vi "General Setting.vi"() -> ()   [LabVIEW 2020, in "Setting Lib.lvlib"]
uses:
  Setting Lib.lvlib
  Database Lib.lvlib
panel:
  in  "Frame Rate":u8=1 min=1 max=5 step=1
  in  "Threshold 5":dbl format="%#.1f"
  in  "Threshold 4":dbl format="%#.1f"
  in  "Threshold 3":dbl format="%#.1f"
  in  "Threshold 2":dbl format="%#.1f"
  in  "Threshold 1":dbl format="%#.1f"
  in  "Close":bool
  # "General Settings"
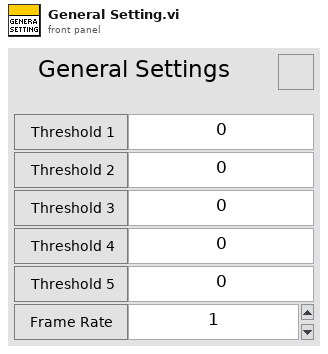
[diagram p1: front panel]
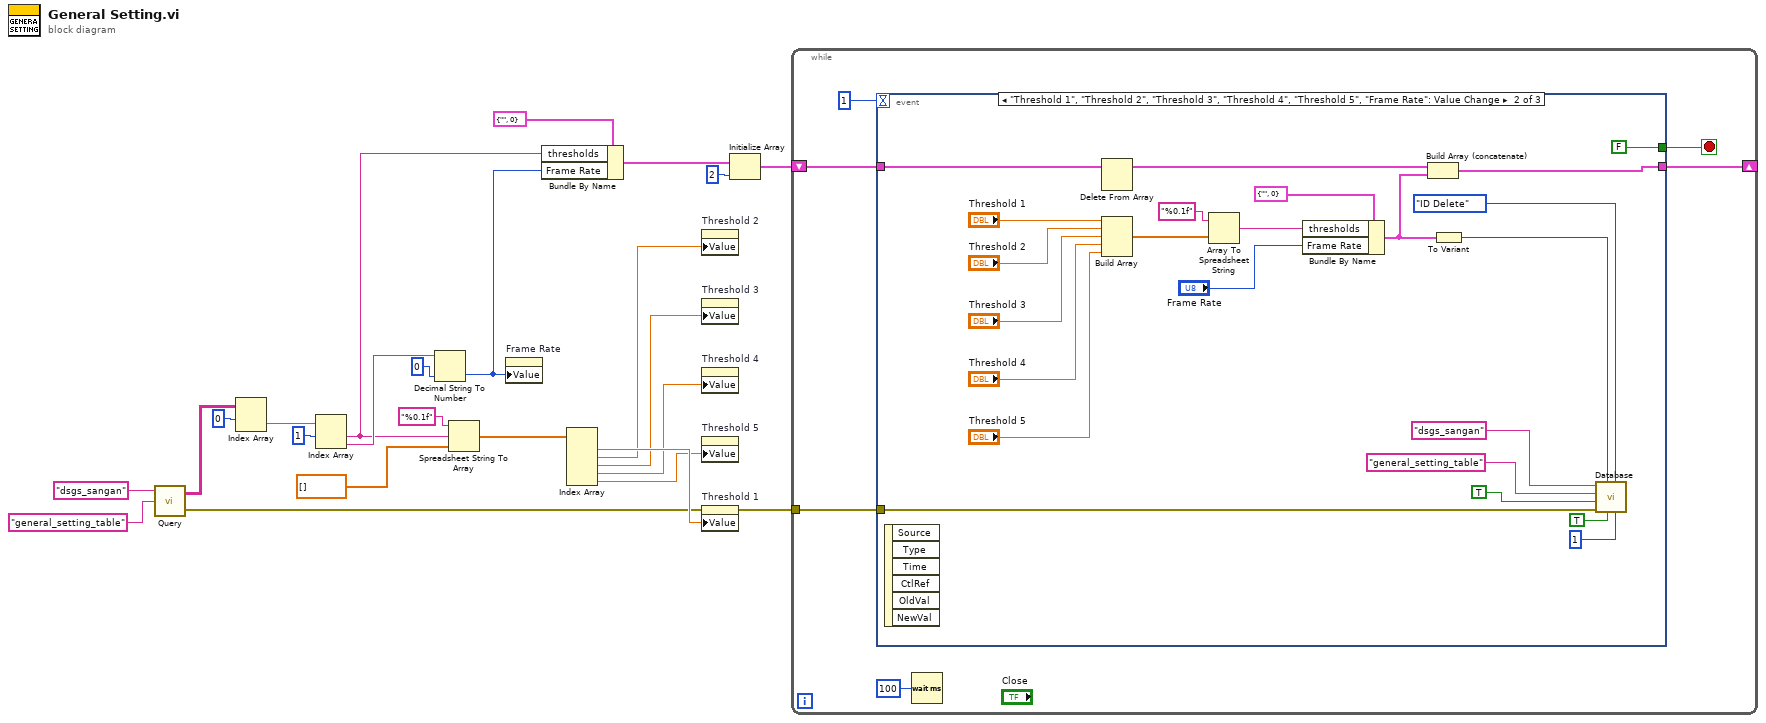
[diagram p0: block diagram]
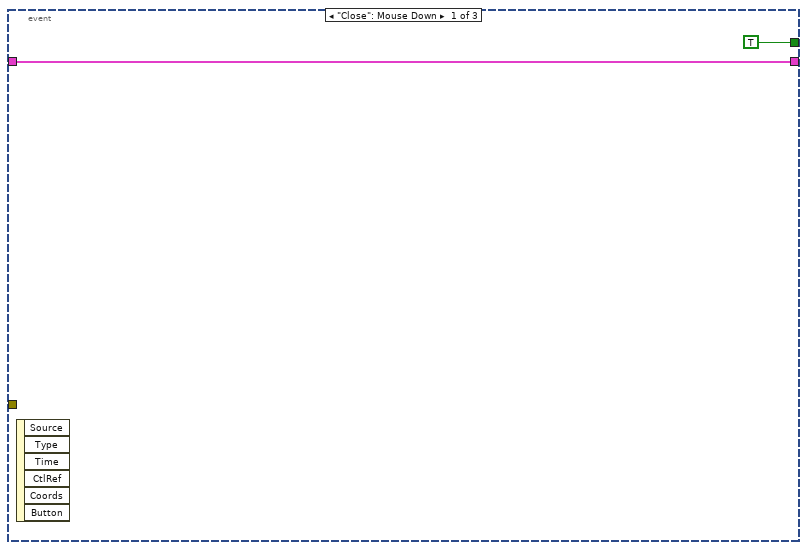
[diagram p2: hidden frame]
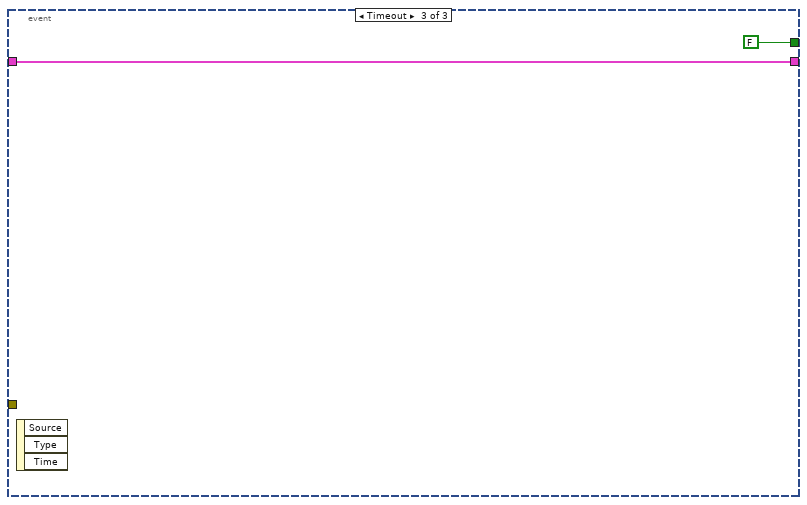
[diagram p3: hidden frame]
diagram:
  n1 = call "Query.vi"("Table Name"="general_setting_table", "Connection Name"="dsgs_sangan") -> ("Error out"=w8:errorcluster, "data"=w22:string[][])  [unwired: 2 in]
  n2 = Index Array(array=w22, index (row)=0) -> (element=w21:string[])  [unwired: 1 in]
  n3 = Index Array(array=w21, index #1=1 ("index")) -> (element #1=w3:string, element #2=w6:string)  [unwired: 1 in]
  n4 = Decimal String To Number(string=w6, default (0L)=u8 0 ("default (0 I32)")) -> (number=w2:u8)  [unwired: 1 in, 1 out]
  n5 = Spreadsheet String To Array(format string="%0.1f", spreadsheet string=w3, array type (2D Dbl)=dbl[] []) -> (array=w15:dbl[])  [unwired: 1 in]
  n6 = property on="Frame Rate" class="DigNum (strict)"("Value"=w2) -> ()  [unwired: 2 in, 2 out]
  n7 = Bundle By Name(cluster=cluster{"thresholds":string, "Frame Rate":u8} {"thresholds"="", "Frame Rate"=0}, "thresholds"=w3, "Frame Rate"=w2) -> (w1:cluster{"thresholds":string, "Frame Rate":u8})
  n8 = Index Array(array=w15) -> (element #1=w13:dbl, element #2=w12:dbl, element #3=w11:dbl, element #4=w10:dbl, element #5=w9:dbl)  [unwired: 5 in]
  n9 = property on="Threshold 2" class="DigNum (strict)"("Value"=w12) -> ()  [unwired: 2 in, 2 out]
  n10 = property on="Threshold 3" class="DigNum (strict)"("Value"=w11) -> ()  [unwired: 2 in, 2 out]
  n11 = property on="Threshold 4" class="DigNum (strict)"("Value"=w10) -> ()  [unwired: 2 in, 2 out]
  n12 = property on="Threshold 5" class="DigNum (strict)"("Value"=w9) -> ()  [unwired: 2 in, 2 out]
  n13 = property on="Threshold 1" class="DigNum (strict)"(error in=w8, "Value"=w13) -> (error out=w7:errorcluster)  [unwired: 1 in, 1 out]
  n14 = Initialize Array(w1, 2 ("dimension size")) -> (w14:cluster{"thresholds":string, "Frame Rate":u8}[])
  n15 = while {
    tunnel: w7 -> [w27]
    shift-right: [w25] -> _
    shift-left: w14 -> [w26]
    stop <- w28 stop-if-true
    n16 = event shown="[1] \"Threshold 1\", \"Threshold 2\", \"Threshold 3\", \"Threshold 4\", \"Threshold 5\", \"Frame Rate\": Value Change" {
      selector: _ -> [_ _ _]
      dyn-events: _ -> [_ _ _]
      timeout: 1 -> [_ _ _]
      tunnel: [TRUE FALSE FALSE] -> w28
      tunnel: w27 -> [_ w39 _]
      tunnel: w26 -> [w31 w38 w56]
      tunnel: [w31 w35 w56] -> w25
      event "Close": Mouse Down {
        n17 = event-data() -> ()  [unwired: 1 in, 6 out]
      }
      event "Threshold 1", "Threshold 2", "Threshold 3", "Threshold 4", "Threshold 5", "Frame Rate": Value Change {
        n18 = event-data() -> ()  [unwired: 1 in, 6 out]
        n19 = Delete From Array(array=w38) -> (array with subset deleted=w37:cluster{"thresholds":string, "Frame Rate":u8}[])  [unwired: 2 in, 1 out]
        n20 = Build Array("Threshold 1", "Threshold 2", "Threshold 3", "Threshold 4", "Threshold 5") -> (w49:dbl[])
        n21 = Array To Spreadsheet String(array=w49, 3:"%0.1f" ("format string")) -> (spreadsheet string=w36:string)  [unwired: 1 in]
        n22 = Bundle By Name(cluster=cluster{"thresholds":string, "Frame Rate":u8} {"thresholds"="", "Frame Rate"=0}, "thresholds"=w36, "Frame Rate"="Frame Rate") -> (w33:cluster{"thresholds":string, "Frame Rate":u8})
        n23 = Build Array (concatenate)(w37, w33) -> (w35:cluster{"thresholds":string, "Frame Rate":u8}[])
        n24 = To Variant(anything=w33) -> (Variant=w42:variant)
        n25 = call "Database.vi"("Maximum Row"=1, "Enum"=enum16{"ID Delete", "Time Delete"}."ID Delete", "Delete row?"=TRUE, "Data"=w42, "Error in"=w39, "Auto Increment ID?"=TRUE, "Table"="general_setting_table", "Connection"="dsgs_sangan") -> ()  [unwired: 3 in, 1 out]
      }
      event Timeout {
        n26 = event-data() -> ()  [unwired: 1 in, 3 out]
      }
    }
    n27 = Wait (ms)(milliseconds to wait=u32 100) -> ()  [unwired: 1 out]
  }
